vi "DAQ@CompareCoverBy__Parameter.vi"(1 "ParamterIn":string) -> (0 "ParamterOut":string)   [LabVIEW 2019]
panel:
  in  "CoverBy":string(combo)
  in  "WaveFormName":string(combo)
  in  "Confirm":bool
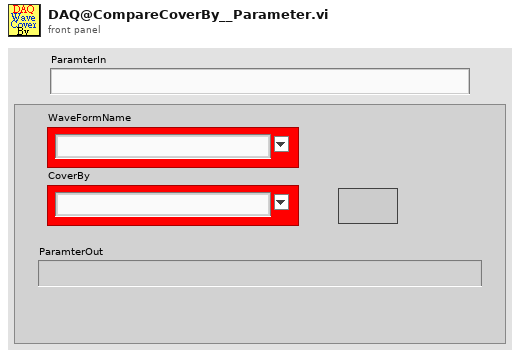
[diagram p1: front panel]
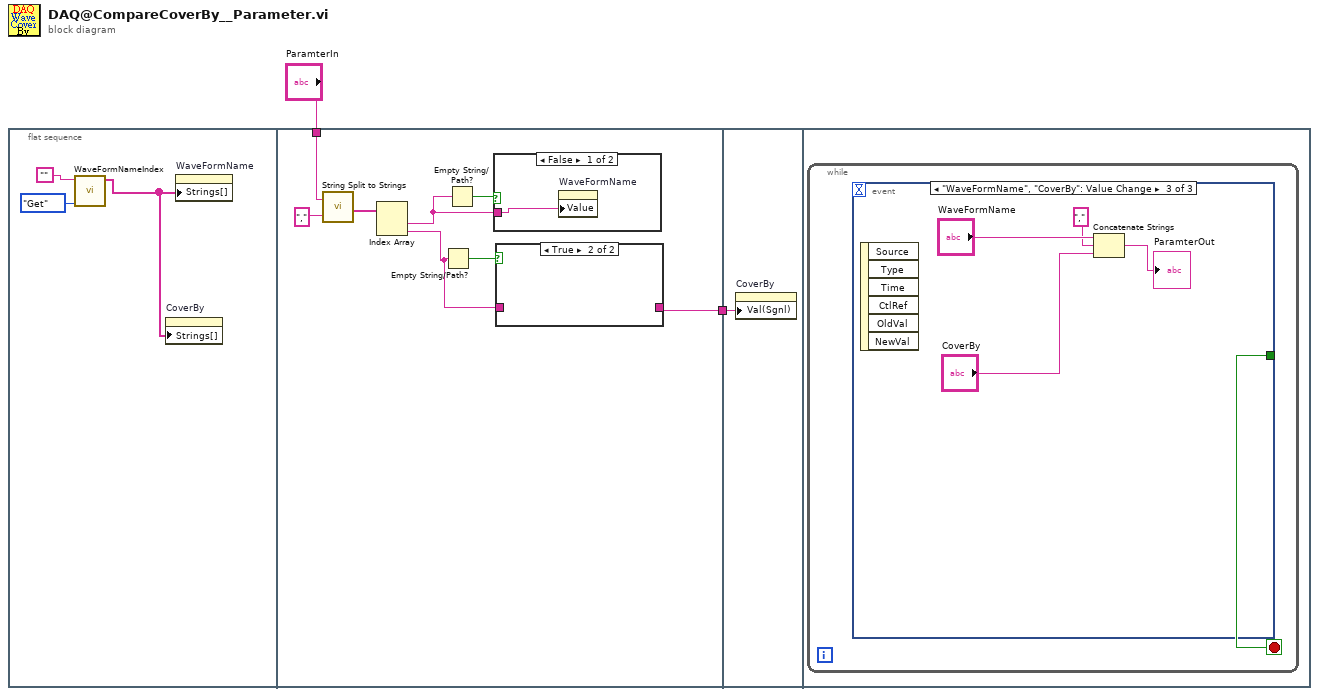
[diagram p0: block diagram]
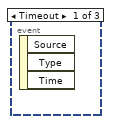
[diagram p4: hidden frame]
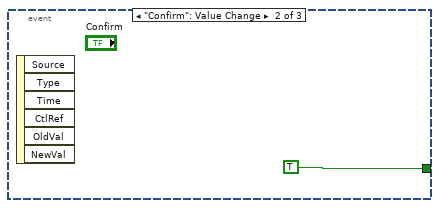
[diagram p5: hidden frame]
diagram:
  n1 = flat-sequence {
    tunnel: "ParamterIn" -> [w11]
    tunnel: [w6] -> w1
    tunnel: w1 -> [w16]
    frame #0 {
      n2 = call "WaveFormNameIndex.vi"("OP"=enum16{"Get", "Update", "Init", "GetSPS"}."Get", "WaveFormName"="") -> ("WaveFormNameList"=w3:string[])  [unwired: 6 in, 3 out]
      n3 = property on="CoverBy" class="CmbBox"("Strings[]"=w3) -> ()  [unwired: 2 in, 2 out]
      n4 = property on="WaveFormName" class="CmbBox"("Strings[]"=w3) -> ()  [unwired: 2 in, 2 out]
    }
    frame #1 {
      n5 = call "String Split to Strings.vi"("search string/char (-)"=",", "String"=w11) -> ("Array"=w10:string[])
      n6 = Index Array(array=w10) -> (element #1=w9:string, element #2=w7:string)  [unwired: 2 in]
      n7 = Empty String/Path?(string/path=w7) -> (empty?=w8:bool)
      n8 = Empty String/Path?(string/path=w9) -> (empty?=w13:bool)
      n9 = case shown="False" w13 {
        tunnel: w9 -> [w15 _]
        frame False {
          n10 = property on="WaveFormName" class="CmbBox"("Value"=w15) -> ()  [unwired: 2 in, 2 out]
        }
        frame True {
        }
      }
      n11 = case shown="True" w8 {
        tunnel: w7 -> [w14 _]
        tunnel: [w14 _] -> w6
        frame False {
        }
        frame True {
        }
      }
    }
    frame #2 {
      n12 = property on="CoverBy" class="CmbBox"("Val(Sgnl)"=w16) -> ()  [unwired: 2 in, 2 out]
    }
    frame #3 {
      n13 = while {
        stop <- w17 stop-if-true
        n14 = event shown="[2] \"WaveFormName\", \"CoverBy\": Value Change" {
          selector: _ -> [_ _ _]
          dyn-events: _ -> [_ _ _]
          timeout: _ -> [_ _ _]
          tunnel: [_ TRUE _] -> w17
          event Timeout {
            n15 = event-data() -> ()  [unwired: 1 in, 3 out]
          }
          event "Confirm": Value Change {
            n16 = event-data() -> ()  [unwired: 1 in, 6 out]
          }
          event "WaveFormName", "CoverBy": Value Change {
            n17 = event-data() -> ()  [unwired: 1 in, 6 out]
            n18 = Concatenate Strings("WaveFormName", ",", "CoverBy") -> (→"ParamterOut":string)
          }
        }
      }
    }
  }
